vi "LWXPS_PositionerPositionComparePulseParametersSet.vi"(0 "XPS Reference IN":refnum<k24>, 5 "Positioner Name":string, 7 "Width of PCO pulses":dbl, 9 "Encoder signal settling time":dbl, 11 "LabVIEW error IN":errorcluster) -> (4 "XPS Reference OUT":refnum<k24>, 6 "Returned error code":i32, 8 "XPS Error String":string, 15 "LabVIEW error OUT":errorcluster)   [LabVIEW 2014]
uses:
  D:/XPSQ8_LabView_Library/Development/Source/Dll/Newport.XPS.CommandInterface.dll
  Dll/Newport.XPS.CommandInterface.dll
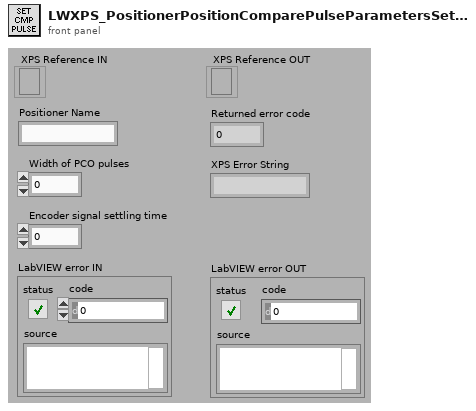
[diagram p1: front panel]
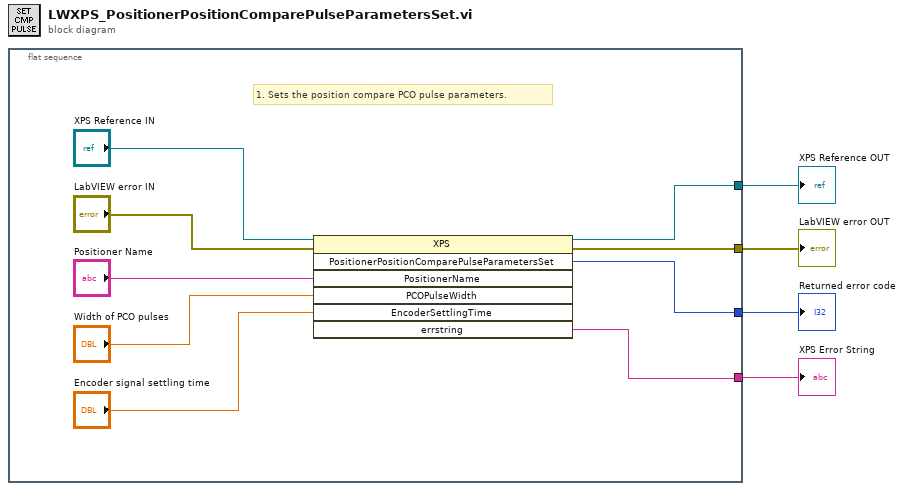
[diagram p0: block diagram]
diagram:
  n1 = flat-sequence {
    tunnel: [w9] -> w4
    tunnel: [w8] -> w3
    tunnel: [w10] -> w2
    tunnel: [w6] -> w1
    frame #0 {
      # "1. Sets the position compare PCO pulse parameters."
      n2 = invoke class="XPS" method="PositionerPositionComparePulseParametersSet"(reference="XPS Reference IN", error in="LabVIEW error IN", "PositionerName"="Positioner Name", "PCOPulseWidth"="Width of PCO pulses", "EncoderSettlingTime"="Encoder signal settling time") -> (reference out=w9:refnum<k24>, error out=w8:errorcluster, "PositionerPositionComparePulseParametersSet"=w10:i32, "errstring"=w6:string)  [unwired: 2 in, 3 out]
    }
  }
  "XPS Error String" <- w1
  "XPS Reference OUT" <- w4
  "LabVIEW error OUT" <- w3
  "Returned error code" <- w2
